vi "NF WF1973_74 AMPL Unit.vi"(6 "Read(F)":bool, 8 "error in (no error)":errorcluster caption="Error IN", 10 "Ch(Ch1)":bool, 11 "VISAsession":refnum<visa-resource-name>) -> (0 "error out":errorcluster caption="Error OUT", 2 "Query Unit":string, 3 "CopyVISAsession":refnum<visa-resource-name>)   [LabVIEW 2010]
panel:
  in  "Unit(Vpp)":u16(ring) items=["Vpp", "Vpk", "Vrms", "dBv", "dBm", "User"]
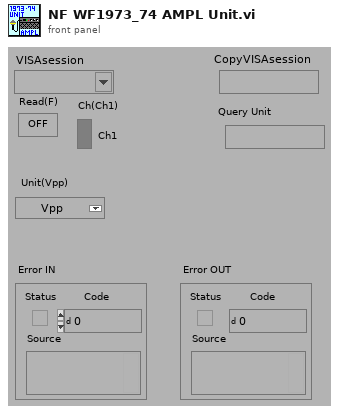
[diagram p1: front panel]
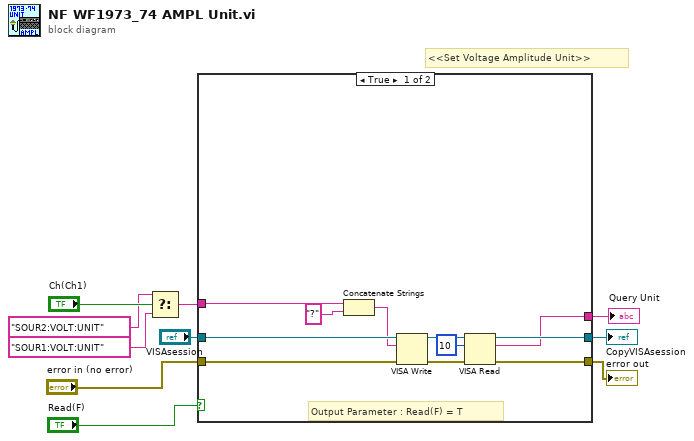
[diagram p0: block diagram]
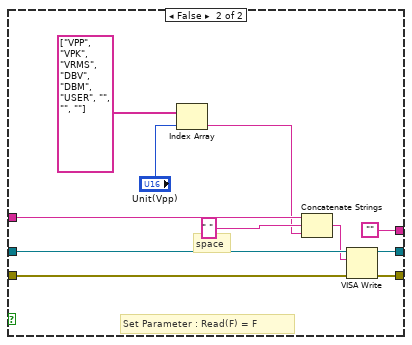
[diagram p2: hidden frame]
diagram:
  # "<<Set Voltage Amplitude Unit>>"
  n1 = Select(t="SOUR2:VOLT:UNIT" ("文字列"), s="Ch(Ch1)", f="SOUR1:VOLT:UNIT" ("文字列")) -> (s? t:f=w3:string)
  n2 = case shown="TRUE" "Read(F)" {
    tunnel: "VISAsession" -> [w21 w32]
    tunnel: [w18 w30] -> w9
    tunnel: [w17 w31] -> w8
    tunnel: "error in (no error)" -> [w16 w26]
    tunnel: w3 -> [w14 w27]
    tunnel: [w11 ""] -> w5
    frame True {
      # "Output Parameter : Read(F) = T"
      n3 = Concatenate Strings(w14, "?" ("形式文字列")) -> (w12:string)
      n4 = VISA Write(VISA resource name=w21, write buffer=w12, error in (no error)=w16) -> (VISA resource name out=w19:refnum<visa-resource-name>, error out=w20:errorcluster)  [unwired: 1 out]
      n5 = VISA Read(VISA resource name=w19, byte count=u32 10 ("バイトカウント（0）"), error in (no error)=w20) -> (VISA resource name out=w18:refnum<visa-resource-name>, read buffer=w11:string, error out=w17:errorcluster)  [unwired: 1 out]
    }
    frame False {
      # "space"
      # "Set Parameter : Read(F) = F"
      n6 = Index Array(array=string[] ["VPP", "VPK", "VRMS", "DBV", "DBM", "USER", "", "", ""], index="Unit(Vpp)") -> (element=w22:string)
      n7 = Concatenate Strings(w27, " ", w22) -> (w29:string)
      n8 = VISA Write(VISA resource name=w32, write buffer=w29, error in (no error)=w26) -> (VISA resource name out=w30:refnum<visa-resource-name>, error out=w31:errorcluster)  [unwired: 1 out]
    }
  }
  "error out" <- w8
  "CopyVISAsession" <- w9
  "Query Unit" <- w5
